vi "Potting Data - HDI Pad Groups.vi"(8 "error in":errorcluster, 9 "Config Manager":refnum<class "Config Manager Class.lvclass">, 10 "Potting Selection HDI Bond Pads":bool[](array[boolean]), 11 "HDI Bond Pad References":T2[](array[typedef])) -> (0 "error out":errorcluster, 3 "Potting Lines":T1[](array[typedef]))   [LabVIEW 2011]
uses:
  Shared Components/Utils/Type Definitions/Fiducial Image.ctl
  Shared Components/Vec3d Class/Vec3d Class.lvclass
  Shared Components/Utils/Type Definitions/Physical Image.ctl
  <vilib>/vision/Image Controls.llb/IMAQ Image.ctl
  Shared Components/Utils/Type Definitions/Fiducial with Source.ctl
  Shared Components/Config Manager Class/Config Manager Class.lvclass
  Shared Components/Utils/Type Definitions/3d Line.ctl
  Shared Components/Config Manager Class/Type Definitions/Part Type.ctl
  Shared Components/Config Manager Class/Read Geometry Definition Integer.vi
  Shared Components/Config Manager Class/Read Geometry Definition Double.vi
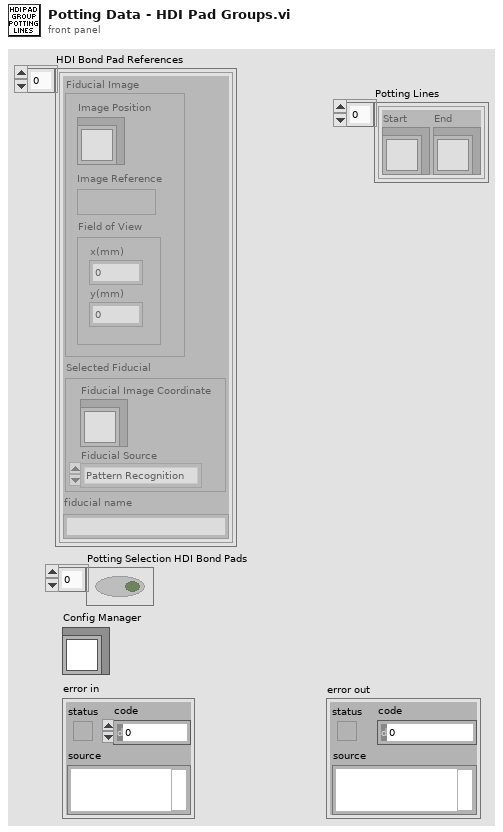
[diagram p1: front panel]
types:
  T1 = typedef "3d Line.ctl" = cluster{"Start":refnum<class "Vec3d Class.lvclass">, "End":refnum<class "Vec3d Class.lvclass">}
  T2 = typedef "Fiducial Image.ctl" = cluster{"Fiducial Image":T3, "Selected Fiducial":T5, "fiducial name":string}
  T3 = typedef "Physical Image.ctl" = cluster{"Image Position":refnum<class "Vec3d Class.lvclass">, "Image Reference":T4, "Field of View":cluster{"x(mm)":dbl, "y(mm)":dbl}}
  T4 = typedef "IMAQ Image.ctl" = refnum<image>
  T5 = typedef "Fiducial with Source.ctl" = cluster{"Fiducial Image Coordinate":refnum<class "Vec3d Class.lvclass">, "Fiducial Source":enum16{"Pattern Recognition", "User", "Error", "Default"}}
  T6 = typedef "Part Type.ctl" = enum16{"BBM", "HDI", "GLUERESERVOIR", "STAMP", "WEIGHT"}
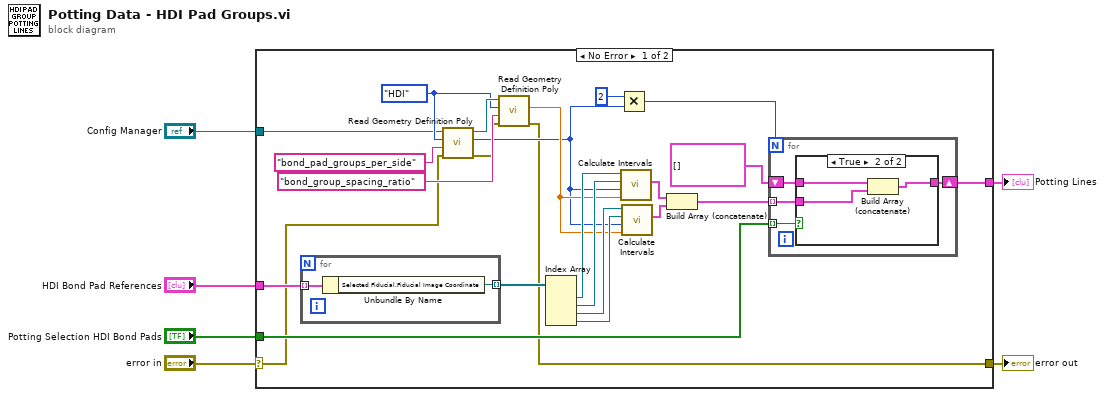
[diagram p0: block diagram]
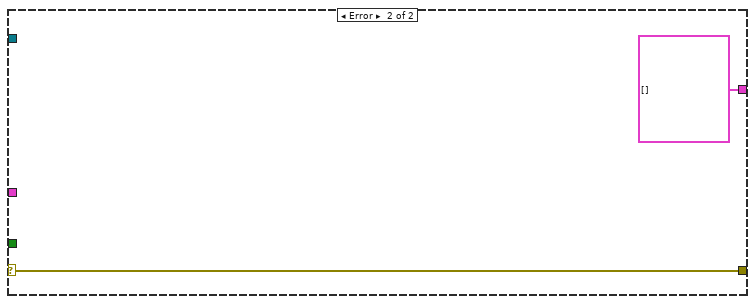
[diagram p3: hidden frame]
diagram:
  n1 = case shown="No Error" "error in" {
    selector: "error in" -> [w9 w42]
    tunnel: "Config Manager" -> [w26 _]
    tunnel: "HDI Bond Pad References" -> [w25 _]
    tunnel: "Potting Selection HDI Bond Pads" -> [w15 _]
    tunnel: [w10 T1[] [] ("appended array")] -> w2
    tunnel: [w7 w42] -> w1
    frame No Error {
      w29 = Part_Type."HDI" ("Part Type")
      n2 = for {
        tunnel: w25 -> [w40] mode=indexing
        tunnel: [w39] -> w24 mode=indexing
        n3 = Unbundle By Name(w40) -> ("Selected Fiducial.Fiducial Image Coordinate"=w39:refnum<class "Vec3d Class.lvclass">)
      }
      n4 = call-poly "Read Geometry Definition Poly.vi"("error in"=w9, "Feature"="bond_pad_groups_per_side", "Part Type"=w29, "Config Manager in"=w26) -> ("error out"=w8:errorcluster, "Geometry Definition"=w13:i32, "Config Manager out"=w30:refnum<class "Config Manager Class.lvclass">)  [unwired: 5 in]
      n5 = call-poly "Read Geometry Definition Poly.vi"("error in"=w8, "Feature"="bond_group_spacing_ratio", "Part Type"=w29, "Config Manager in"=w30) -> ("error out"=w7:errorcluster, "Geometry Definition"=w19:dbl)  [unwired: 5 in, 1 out]
      n6 = Index Array(array=w24) -> (element #1=w23:refnum<class "Vec3d Class.lvclass">, element #2=w22:refnum<class "Vec3d Class.lvclass">, element #3=w21:refnum<class "Vec3d Class.lvclass">, element #4=w20:refnum<class "Vec3d Class.lvclass">)  [unwired: 4 in]
      n7 = Multiply(x=2, y=w13) -> (x*y=w11:i32)
      n8 = call "Calculate Intervals.vi"("gap/group ratio"=w19, "Num Intervals"=w13, "End"=w22, "Start"=w23) -> ("Intervals"=w18:T1[])  [unwired: 7 in]
      n9 = call "Calculate Intervals.vi"("gap/group ratio"=w19, "Num Intervals"=w13, "End"=w20, "Start"=w21) -> ("Intervals"=w17:T1[])  [unwired: 7 in]
      n10 = Build Array (concatenate)(w18, w17) -> (w16:T1[])
      n11 = for {
        N: w11 -> [_]
        tunnel: w16 -> [w32] mode=indexing
        tunnel: w15 -> [w34] mode=indexing
        shift-right: [w31] -> w10
        shift-left: T1[] [] ("appended array") -> [w33]
        n12 = case shown="True" w34 {
          tunnel: w33 -> [w35 w38]
          tunnel: w32 -> [_ w37]
          tunnel: [w35 w36] -> w31
          frame False {
          }
          frame True {
            n13 = Build Array (concatenate)(w38, w37) -> (w36:T1[])
          }
        }
      }
    }
    frame Error {
    }
  }
  "Potting Lines" <- w2
  "error out" <- w1
